vi "2023_day05_Task2_old.vi"() -> ()   [LabVIEW 2021]
panel:
  out "Number of Seeds":i64 format="%_6p"
  out "size(s)":i32
  out "Task 2 (min location)":i64
  in  "Switch":bool caption="Ex. Data  vs.  User Data"
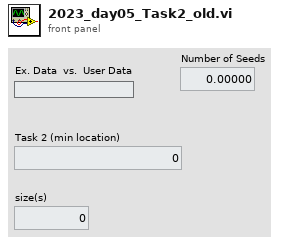
[diagram p1: front panel]
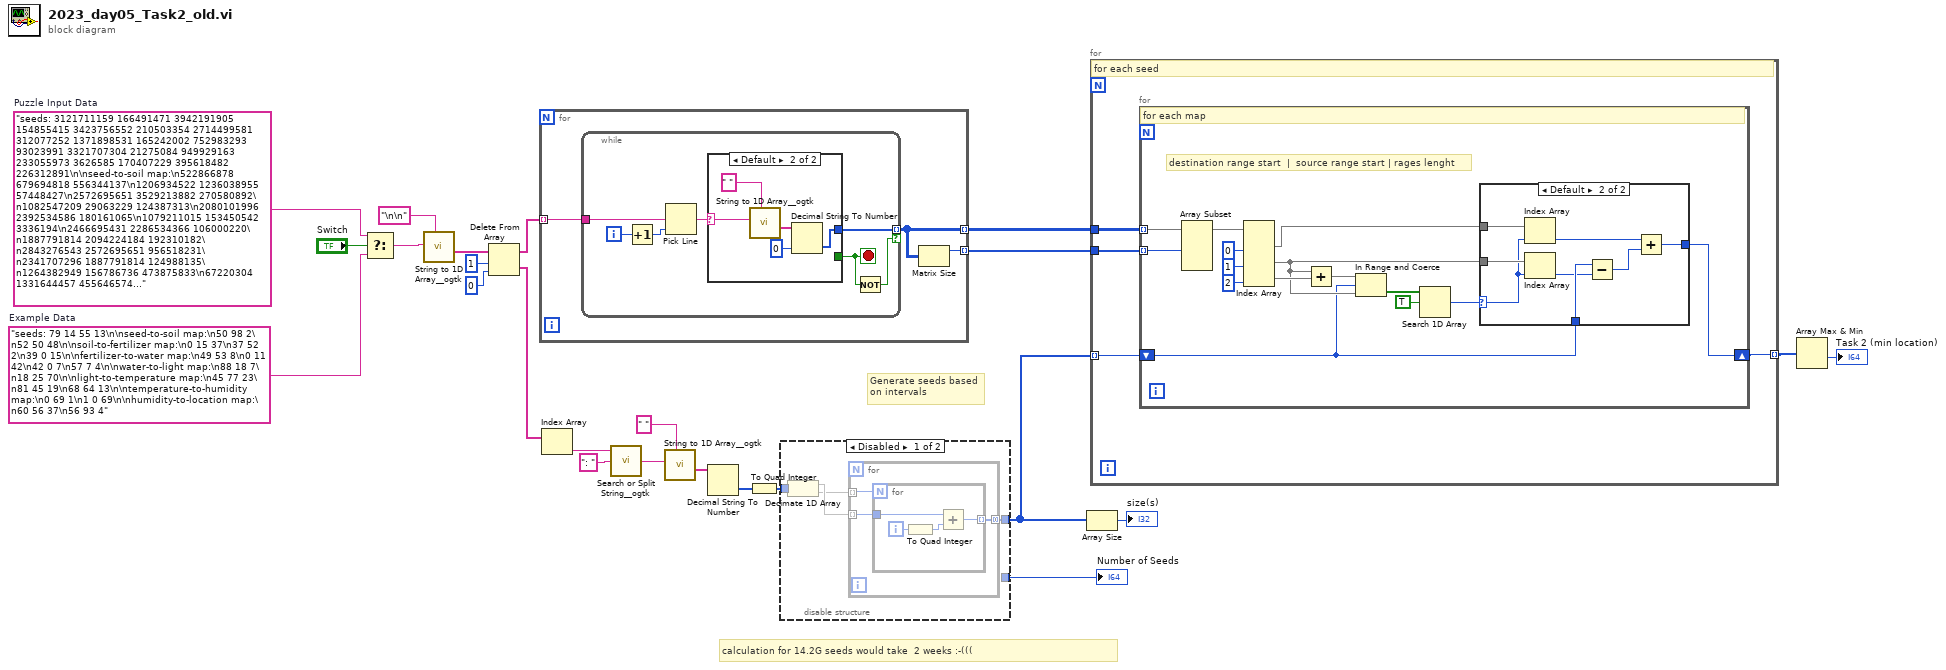
[diagram p0: block diagram]
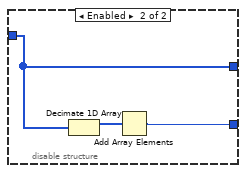
[diagram p2: hidden frame]
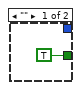
[diagram p3: hidden frame]
diagram:
  w22 = "seeds: 3121711159 166491471 3942191905 154855415 3423756552 210503354 2714499581 312077252 1371898531 165242002 752983293 93023991 3321707304 21275084 949929163 233055973 3626585 170407229 395618482 226312891\n\nseed-to-soil map:\n522866878 679694818 556344137\n1206934522 1236038955 57448427\n2572695651 3529213882 270580892\n1082547209 29063229 124387313\n2080101996 2392534586 180161065\n1079211015 153450542 3336194\n2466695431 2286534366 106000220\n1887791814 2094224184 192310182\n2843276543 2572695651 956518231\n2341707296 1887791814 124988135\n1264382949 156786736 473875833\n67220304 1331644457 455646574\n3903217571 3799794774 267521683\n2260263061 2012779949 81444235\n1738258782 630662569 49032249\n29063229 1293487382 38157075\n3799794774 4067316457 103422797\n\nsoil-to-fertilizer map:\n69994133 1665188283 300635345\n0 1965823628 36826481\n2222587532 2553838094 476943506\n2929387922 3030781600 856348250\n4182440411 2441311209 112526885\n36826481 2002650109 33167652\n2044606970 4116986734 177980562\n1815516279 549395220 220301482\n1186435707 0 549395220\n916609638 1315676862 269826069\n3785736172 2044606970 396704239\n2699531038 3887129850 229856884\n1735830927 1585502931 79685352\n370629478 769696702 545980160\n\nfertilizer-to-water map:\n2485494684 3430237839 78539769\n2045426403 2253341567 99573285\n290571869 0 280695139\n3540352207 2045426403 63912525\n2879366909 3356847577 67075608\n868611408 858081124 224160766\n2304858397 2525185867 55003581\n189640733 280695139 100931136\n2144999688 3983682880 159858709\n3374818325 3858616265 14108175\n3604264732 2580189448 427645906\n1730244179 535856806 2894582\n4242091162 3634410314 52876134\n4031910638 3872724440 110958440\n1092772174 1116784935 90115688\n1182887862 381626275 154230531\n4149183732 3263940147 92907430\n4142869078 3423923185 6314654\n571267008 728392121 129689003\n3315918322 2352914852 58900003\n2359861978 3508777608 125632706\n2735364270 2109338928 144002639\n2946442517 2411814855 113371012\n1733138761 1082241890 34543045\n700956011 1600026409 167655397\n3059813529 3041876971 222063176\n2564034453 3687286448 171329817\n3281876705 3007835354 34041617\n0 538751388 189640733\n3388926500 4143541589 151425707\n1337118393 1206900623 393125786\n\nwater-to-light map:\n66525849 932008802 34502691\n1231709999 161981088 108836128\n4050378444 3046032039 195065028\n1188304980 324179540 43405019\n0 95455239 66525849\n1134942656 270817216 53362324\n4015087939 2401779423 35290505\n3174436586 2144628864 257150559\n3688283374 3968162731 326804565\n101028540 367584559 564424243\n665452783 23428765 72026474\n2144628864 2437069928 302742058\n1340546127 0 23428765\n737479257 1714174561 397463399\n3431587145 2789335810 256696229\n4245443472 2739811986 49523824\n1363974892 966511493 747663068\n2447370922 3241097067 727065664\n\nlight-to-temperature map:\n3188351957 4202865263 58820659\n583430260 717912118 192120954\n1044551258 2246397764 71032709\n3109547837 4261685922 33281374\n1678878772 1586709546 87694921\n1115583967 3604496785 152969541\n3142829211 2200875018 45522746\n2103724421 1412959073 173750473\n3094755823 2836912864 14792014\n4233716778 2851704878 61250518\n1809783323 3254776949 293941098\n570222212 2097755032 13208048\n34744215 693464 72237295\n1773265141 2502078476 36518182\n775551214 4072807084 98261716\n2718819720 511651563 117721319\n873812930 4171068800 31796463\n905609393 3933865219 138941865\n373474927 3892288779 41576440\n3040218555 3117948789 54537268\n2397118702 2538596658 1887839\n0 72930759 34744215\n2277474894 1316613368 93303271\n370955311 1409916639 2519616\n1359408316 3757466326 134822453\n2370778165 306806837 1167210\n220512052 1412436255 522818\n3335711852 1674404467 423350565\n335173455 2743397480 35781856\n3900016435 982913025 333700343\n2399006541 2540484497 202912983\n3816795945 2110963080 83220490\n415051367 910033072 72879953\n2663040982 3548718047 55778738\n3759062417 2779179336 57733528\n3247172616 629372882 88539236\n1494230769 2317430473 184648003\n1766573693 2194183570 6691448\n2601919524 245685379 61121458\n2371945375 220512052 25173327\n221034870 3003810204 114138585\n2836541039 307974047 203677516\n487931320 3172486057 82290892\n106981510 0 693464\n1268553508 2912955396 90854808\n\ntemperature-to-humidity map:\n1844491325 2716144828 118858329\n1004942401 2971501799 229549152\n696973964 238546929 19842755\n716816719 119302258 119244671\n444146335 2339344684 80152617\n3752420807 853580623 112964826\n3736479208 2933101125 15941599\n1822411864 805752927 11014046\n3183816206 2835003157 98097968\n3538508914 2576089466 88076349\n1833425910 816766973 11065415\n3865385633 2664165815 51979013\n1706894195 1592117663 89769434\n2892814110 3354360228 291002096\n2450334080 3645362324 65003481\n3934652728 3721018678 66888233\n3285923313 2419497301 85776839\n3917364646 2257358228 17288082\n3371700152 2090549466 166808762\n524298952 633077915 172675012\n1600852292 966545449 106041903\n2283983708 620036820 13041095\n2176983704 2274646310 64698374\n2515337561 1072587352 32448957\n846714263 1105036309 42935019\n3719859664 603417276 16619544\n2547786518 258389684 345027592\n0 1147971328 444146335\n1963349654 3787906911 213634050\n836061390 3710365805 10652873\n889649282 0 115293119\n2241682078 1681887097 42301630\n3281914174 115293119 4009139\n2297024803 3201050951 153309277\n1796663629 827832388 25748235\n3626585263 2505274140 70815326\n1234491553 1724188727 366360739\n3697400589 2949042724 22459075\n\nhumidity-to-location map:\n3693038281 1946208152 169064741\n3025397429 1673895501 272312651\n2522027478 1111558812 503369951\n3862103022 3729735566 432864274\n1111558812 2115272893 1374715990\n3356676818 3489988883 239746683\n3297710080 1614928763 58966738\n2486274802 4162599840 35752676\n3596423501 4198352516 96614780"  # Puzzle Input Data
  w23 = "seeds: 79 14 55 13\n\nseed-to-soil map:\n50 98 2\n52 50 48\n\nsoil-to-fertilizer map:\n0 15 37\n37 52 2\n39 0 15\n\nfertilizer-to-water map:\n49 53 8\n0 11 42\n42 0 7\n57 7 4\n\nwater-to-light map:\n88 18 7\n18 25 70\n\nlight-to-temperature map:\n45 77 23\n81 45 19\n68 64 13\n\ntemperature-to-humidity map:\n0 69 1\n1 0 69\n\nhumidity-to-location map:\n60 56 37\n56 93 4"  # Example Data
  # "calculation for 14.2G seeds would take  2 weeks :-((("
  # "Generate seeds based\non intervals"
  n1 = Select(t=w22, s="Switch", f=w23) -> (s? t:f=w21:string)
  n2 = call <userlib>:"String to 1D Array__ogtk.vi"("delimiter (Tab)"="\n\n", "string"=w21) -> ("Array of Strings"=w19:string[])  [unwired: 9 in]
  n3 = Delete From Array(array=w19, length=1, index=0) -> (deleted portion=w16:string[], array with subset deleted=w11:string[])
  n4 = for {
    tunnel: w11 -> [w27] mode=indexing
    tunnel: [w26] -> w6 mode=indexing
    tunnel: [w25] -> w5 mode=indexing
    n5 = while {
      tunnel: w27 -> [w34]
      tunnel: [w28] -> w26 mode=indexing if=w29
      i -> [w33]
      stop <- w30 stop-if-true
      n6 = Increment(x=w33) -> (x+1=w32:i32)
      n7 = Pick Line(multi-line string=w34, line index=w32) -> (output string=w31:string)  [unwired: 1 in]
      n8 = case shown="Default" w31 {
        selector: w31 -> [_ w39]
        tunnel: [TRUE _] -> w30
        tunnel: [_ w37] -> w28
        frame "" {
        }
        frame Default {
          n9 = call <userlib>:"String to 1D Array__ogtk.vi"("delimiter (Tab)"=" ", "string"=w39) -> ("Array of Strings"=w38:string[])  [unwired: 9 in]
          n10 = Decimal String To Number(string=w38, default (0L)=i64 0 ("default (0 I32)")) -> (number=w37:i64[])  [unwired: 1 in, 1 out]
        }
      }
      n11 = Not(x=w30) -> (.not. x?=w29:bool)
    }
    n12 = Matrix Size(0:w26) -> (1:w25:i32)  [unwired: 1 out]
  }
  n13 = Index Array(array=w16) -> (element=w15:string)  [unwired: 1 in]
  n14 = call <userlib>:"Search or Split String__ogtk.vi"("search string/char (-)"=": ", "string"=w15) -> ("substring after match"=w13:string)  [unwired: 1 in, 2 out]
  n15 = call <userlib>:"String to 1D Array__ogtk.vi"("delimiter (Tab)"=" ", "string"=w13) -> ("Array of Strings"=w10:string[])  [unwired: 9 in]
  n16 = Decimal String To Number(string=w10) -> (number=w7:i32[])  [unwired: 2 in, 1 out]
  n17 = To Quad Integer(1:w7) -> (0:w3:i64[])
  n18 = disable-structure shown="Disabled" {
    disable-tunnel: w3 -> [w42 w54]
    disable-tunnel: [w41 w54] -> w2
    disable-tunnel: [_ w52] -> w1
    frame Disabled {
      n19 = Decimate 1D Array(w42) -> (w44:i64[], w43:i64[])
      n20 = for {
        tunnel: w44 -> [w46] mode=indexing
        tunnel: w43 -> [w47] mode=indexing
        tunnel: [w45] -> w41 mode=concatenating
        n21 = for {
          N: w47 -> [_]
          tunnel: w46 -> [w51]
          tunnel: [w50] -> w45 mode=indexing
          i -> [w48]
          n22 = To Quad Integer(1:w48) -> (0:w49:i64)
          n23 = Add(x=w51, y=w49) -> (x+y=w50:i64)
        }
      }
    }
    frame Enabled {
      n24 = Decimate 1D Array(w54) -> (w53:i64[])  [unwired: 1 out]
      n25 = Add Array Elements(numeric array=w53) -> (sum=w52:i64)
    }
  }
  "Number of Seeds" <- w1
  n26 = Array Size(array=w2) -> (size(s)=→"size(s)":i32)
  n27 = for {
    tunnel: w2 -> [w58] mode=indexing
    tunnel: w6 -> [w57]
    tunnel: w5 -> [w56]
    tunnel: [w55] -> w9 mode=indexing
    # "for each seed"
    n28 = for {
      tunnel: w57 -> [w73] mode=indexing
      tunnel: w56 -> [w60] mode=indexing
      shift-right: [w62] -> w55
      shift-left: w58 -> [w64]
      # "destination range start  |  source range start | rages lenght"
      # "for each map"
      n29 = Array Subset(array=w73, length (row)=w60) -> (w61:i64[][])  [unwired: 3 in]
      n30 = Index Array(array=w61, index (col) #1=0 ("disabled index (col)"), index (col) #2=1 ("index (col)"), index (col) #3=2 ("index (col)")) -> (element #1=w59:i64[], element #2=w65:i64[], element #3=w69:i64[])  [unwired: 3 in]
      n31 = Add(x=w65, y=w69) -> (x+y=w68:i64[])
      n32 = In Range and Coerce(upper limit=w68, x=w64, lower limit=w65) -> (In Range?=w67:bool[])  [unwired: 1 out]
      n33 = Search 1D Array(1D array=w67, element=TRUE) -> (index of element=w63:i32)  [unwired: 1 in]
      n34 = case shown="Default" w63 {
        selector: w63 -> [_ w79]
        tunnel: w65 -> [_ w82]
        tunnel: w64 -> [w74 w81]
        tunnel: w59 -> [_ w78]
        tunnel: [w74 w75] -> w62
        frame -1 {
        }
        frame Default {
          n35 = Index Array(array=w78, index=w79) -> (element=w76:i64)
          n36 = Index Array(array=w82, index=w79) -> (element=w80:i64)
          n37 = Subtract(x=w81, y=w80) -> (x-y=w77:i64)
          n38 = Add(x=w76, y=w77) -> (x+y=w75:i64)
        }
      }
    }
  }
  n39 = Array Max & Min(array=w9) -> (min value=→"Task 2 (min location)":i64)  [unwired: 3 out]
